vi "_Update Start Up Turbo.vi"(4 "error in (no error)":errorcluster) -> (0 "error Out":errorcluster, 2 "Next InstrState":T1, 3 "Cancel":bool)   [LabVIEW 2018]
uses:
  Type/_RT Instrument State.ctl
  Type/_Pump Parameter.ctl
  Type/_LCD Line1 Msg.ctl
  Type/_LCD Line2 Msg.ctl
  Type/_RW Status.ctl
  Type/_LED States.ctl
  _RT Global.vi
  <vilib>/Utility/error.llb/Error Cluster From Error Code.vi
  <vilib>/rvi/errors/niLvFpgaAdjustHostInterfaceError.vi
  <vilib>/rvi/interface/nirviReadWriteControl/nirviReadWriteControl.xnode
  Type/FPGA Typedef.ctl
  FPGA Bitfiles/FPGA9607.lvbitx
  NiFpgaLv.dll
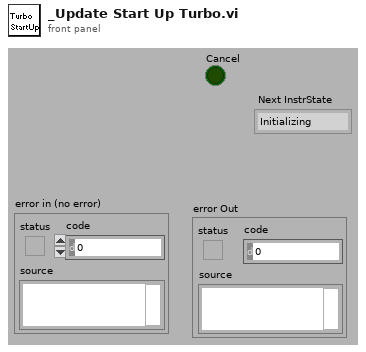
[diagram p1: front panel]
types:
  T1 = typedef "_RT Instrument State.ctl" = enum16{"Initializing", "Mass Spectrometer is Off", "Starting Up", "Turning Power Off", "Going to Standby", "Roughing Pump Ready", "Turning Turbo Off", "Turbo Startup", "Turbopump Ready", "Checking Vacuum", "Going to Ready", "Ready", "Running", "Source Standby", "Lost Communication", "Shutting Down", "Fault", "24V Standby", "Go to 24V Standby", "Turbopump Ready-Waiting"}
  T2 = typedef "_Pump Parameter.ctl" = enum16{"Turn Pump Motor On", "Turn Pump Motor Off", "Read Pump Oil Deficiency", "Read Rotation Switch Point Attained", "Read Ele. Drive Over Temperature", "Read Pump Over Temperature", "Read Set Rotation Speed Attained", "Read Turbopump Accelerates", "Read Actual Rotation Speed in Hz", "Read Motor Current in A", "Read Operating Hours in h", "Read Motor Voltage in V", "Read Motor Power in W", "Set Rotation Speed Switchpoint in %", "Clear Error", "Read Error Code", "Read Bearing Temperature", "Read Hardware Version", "Read Firmware Version", "Read Operating Hours (Drive)", "Read Rotational Speed (rpm)", "Read Power Stage Temperature", "Read Electronics Temperature", "Read Upper Pump Temperature", "Read Motor Temperature", "Read Error Code History, 1", "Read Error Code History, 2", "Read Error Code History, 3", "Read Error Code History, 4", "Read Error Code History, 5", "Read Error Code History, 6", "Read Error Code History, 7", "Read Error Code History, 8", "Read Error Code History, 9", "Read Error Code History, 10"}
  T3 = typedef "_RW Status.ctl" = enum8{"Done", "Do Read", "Do Write", "Set Latch1", "Set Latch2", "Set Latch3", "Set Latch4", "RP ON", "EL ON", "Serial Send", "Set LC Out", "Get LC In", "Read VAC", "Table Test", "Get Interlock", "Do Read2", "Do Write2"}
  T4 = typedef "_LED States.ctl" = enum8{"Idle", "Solid B", "Solid R", "Solid P", "Off B", "Off R", "Off P", "Off BRP", "Off RP", "Flash R&P", "Flash P"}
  T5 = typedef "_LCD Line2 Msg.ctl" = u16
  T6 = typedef "_LCD Line1 Msg.ctl" = u16
  T7 = typedef "_RT Startup Options.ctl" = cluster{"Door":bool, "Curtain":bool, "Pressure":bool, "Turbo":bool, "SysPoll":bool, "GasFlag":bool, "SourceExhaust":bool}
  T8 = typedef "FPGA Typedef.ctl" = refnum<k20>
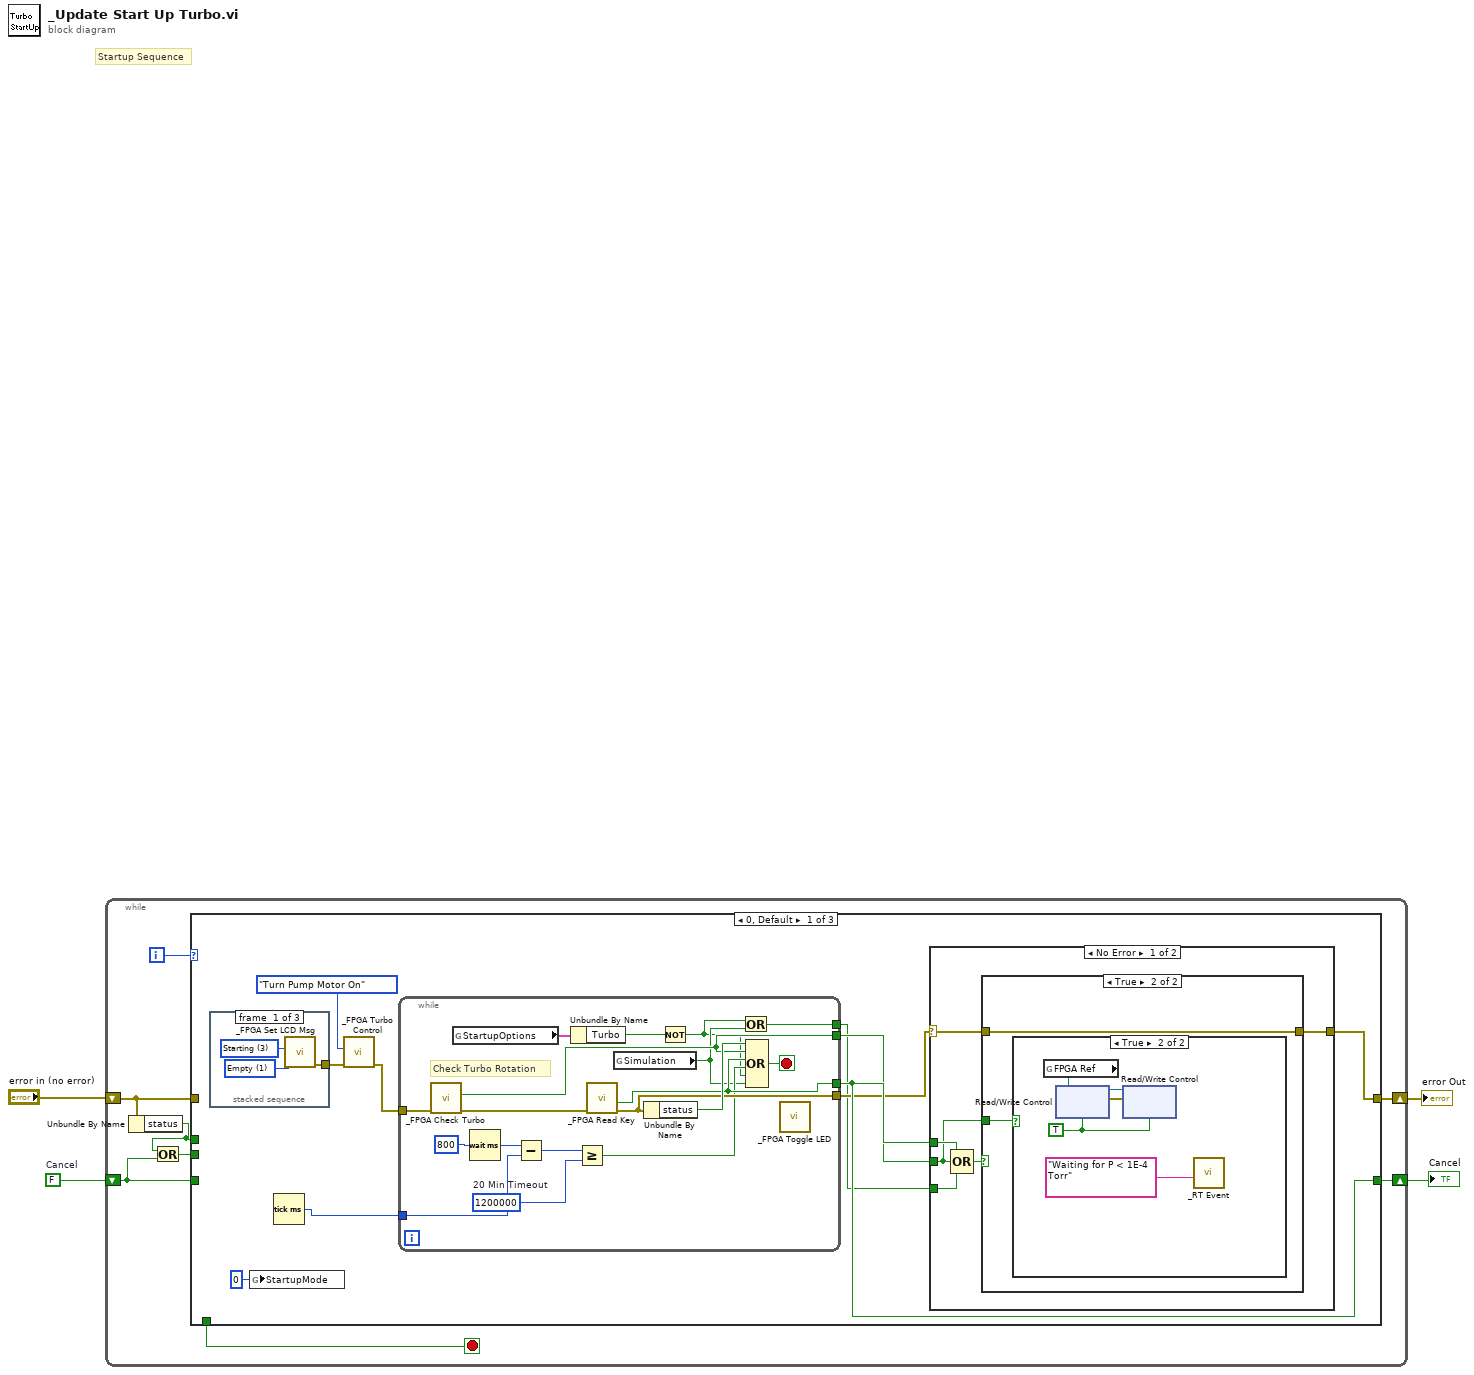
[diagram p0: block diagram]
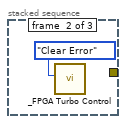
[diagram p2: hidden frame]
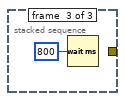
[diagram p3: hidden frame]
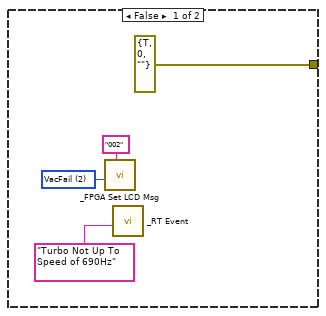
[diagram p4: hidden frame]
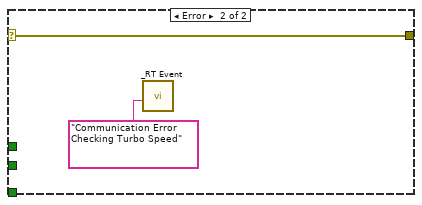
[diagram p6: hidden frame]
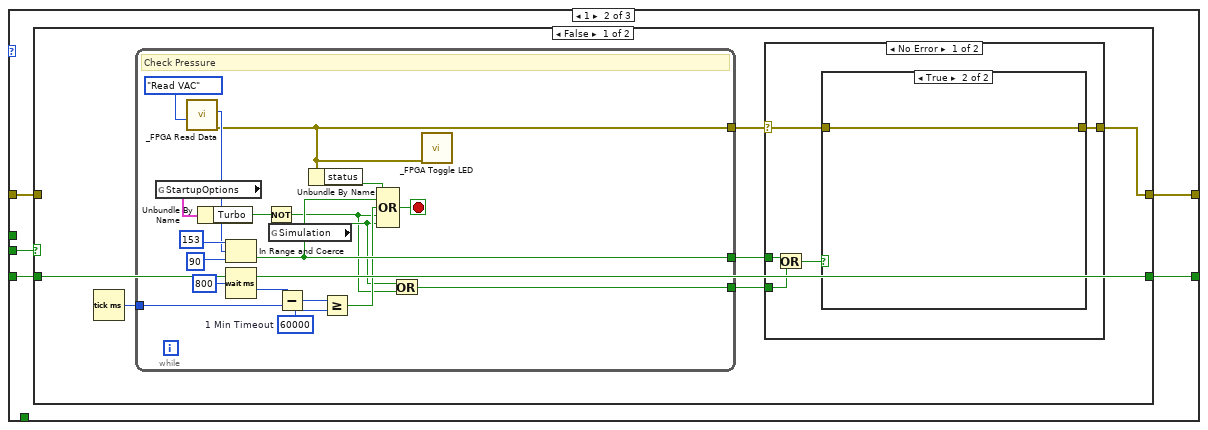
[diagram p7: hidden frame]
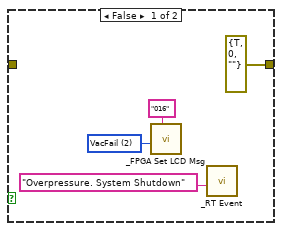
[diagram p8: hidden frame]
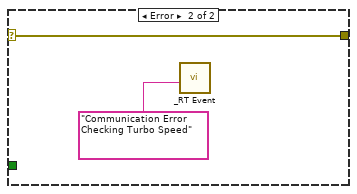
[diagram p9: hidden frame]
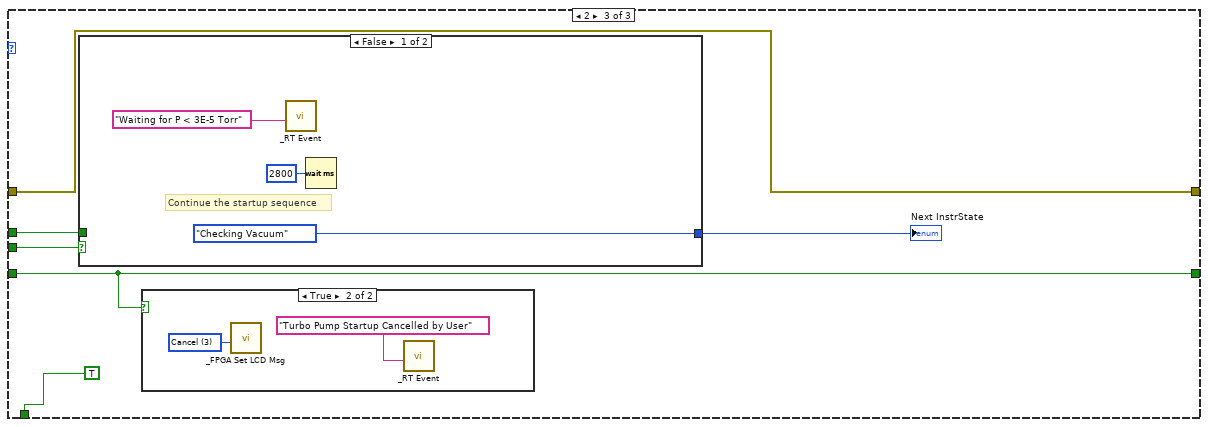
[diagram p11: hidden frame]
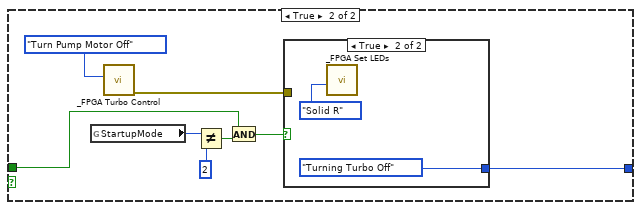
[diagram p12: hidden frame]
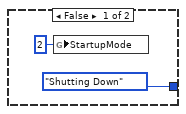
[diagram p13: hidden frame]
diagram:
  w3 = FALSE  # Cancel
  # "Startup Sequence"
  n1 = while {
    shift-right: [w8] -> w2
    shift-left: "error in (no error)" -> [w10]
    shift-right: [w7] -> w1
    shift-left: w3 -> [w9]
    i -> [w12]
    stop <- w6 stop-if-true
    n2 = Unbundle By Name(w10) -> ("status"=w5:bool)
    n3 = Or(x=w5, y=w9) -> (x .or. y?=w11:bool)
    n4 = case shown="0, Default" w12 {
      tunnel: w11 -> [_ w67 w111]
      tunnel: w10 -> [_ w66 w113]
      tunnel: w9 -> [_ w65 w112]
      tunnel: [w22 w69 w113] -> w8
      tunnel: [w21 w68 w112] -> w7
      tunnel: [_ _ TRUE] -> w6
      tunnel: w5 -> [_ _ w109]
      frame 0, Default {
        n5 = stacked-sequence {
          tunnel: [w41 _ _] -> w15
          frame #0 {
            w42 = T5 1 items=["Same", "Empty", "VacFail", "Cancel", "CheckGas", "EleFail", "Probe1Fail", "Probe2Fail", "HeaterFail", "DoorOpen", "CheckComm", "PressStart", "StartRP"] ("Line2Msg (same)")
            w43 = T6 3 items=["Same", "Empty", "Connected", "Starting", "Stopping", "Action", "On", "Service", "Call", "Acquiring", "Source"] ("Line1Msg (same)")
            n6 = call "_FPGA Set LCD Msg.vi"("Line2Msg (same)"=w42, "Line1Msg (same)"=w43) -> ("error out"=w41:errorcluster)  [unwired: 5 in, 2 out]
          }
          frame #1 {
            n7 = call "_FPGA Turbo Control.vi"("Command"=_Pump_Parameter."Clear Error") -> ()  [unwired: 3 in, 6 out]
          }
          frame #2 {
            n8 = Wait (ms)(milliseconds to wait=u32 800) -> ()  [unwired: 1 out]
          }
        }
        n9 = global write "_RT Global.vi" "StartupMode"(u8 0 ("StartupMode")) -> ()
        n10 = Tick Count (ms)() -> (millisecond timer value=w13:u32)
        n11 = call "_FPGA Turbo Control.vi"("error in (no error)"=w15, "Command"=_Pump_Parameter."Turn Pump Motor On") -> ("error out"=w14:errorcluster)  [unwired: 2 in, 5 out]
        n12 = while {
          tunnel: w14 -> [w31]
          tunnel: [w37] -> w20
          tunnel: [w36] -> w21
          tunnel: w13 -> [w32]
          tunnel: [w29] -> w19
          tunnel: [w26] -> w17
          stop <- w40 stop-if-true
          w35 = u32 1200000  # 20 Min Timeout
          # "Check Turbo Rotation"
          n13 = call "_FPGA Check Turbo.vi"("error in"=w31) -> ("error out"=w30:errorcluster, "SpeedOK"=w29:bool)  [unwired: 1 in, 4 out]
          n14 = global read "_RT Global.vi" "StartupOptions"() -> (w25:T7)
          n15 = Wait (ms)(milliseconds to wait=u32 800) -> (millisecond timer value=w33:u32)
          n16 = Subtract(x=w33, y=w32) -> (x-y=w34:u32)
          n17 = Unbundle By Name(w25) -> ("Turbo"=w24:bool)
          n18 = Greater Or Equal?(x=w34, y=w35) -> (x >= y?=w28:bool)
          n19 = call "_FPGA Read Key.vi"("error in (no error)"=w30) -> ("error out"=w37:errorcluster, "Key Pressed"=w36:bool)  [unwired: 3 in, 3 out]
          n20 = global read "_RT Global.vi" "Simulation"() -> (w27:bool)
          n21 = Unbundle By Name(w37) -> ("status"=w39:bool)
          n22 = Not(x=w24) -> (.not. x?=w23:bool)
          n23 = Or(x=w23, y=w27) -> (x .or. y?=w26:bool)
          n24 = Compound Arithmetic op=OR(w39, w29, w36, w28, w23, w27) -> (w40:bool)
          n25 = call "_FPGA Toggle LED.vi"() -> ()  [unwired: 5 in, 4 out]
        }
        n26 = case shown="No Error" w20 {
          selector: w20 -> [w51 w64]
          tunnel: w19 -> [w47 _]
          tunnel: [w50 w64] -> w22
          tunnel: w21 -> [w48 _]
          tunnel: w17 -> [w46 _]
          frame No Error {
            n27 = Compound Arithmetic op=OR(w48, w47, w46) -> (w49:bool)
            n28 = case shown="True" w49 {
              tunnel: [errorcluster {"status"=TRUE, "code"=0, "source"=""} ("error IO") w57] -> w50
              tunnel: w51 -> [_ w57]
              tunnel: w47 -> [_ w56]
              frame False {
                w53 = T5 2 items=["Same", "Empty", "VacFail", "Cancel", "CheckGas", "EleFail", "Probe1Fail", "Probe2Fail", "HeaterFail", "DoorOpen", "CheckComm", "PressStart", "StartRP"] ("Line2Msg (same)")
                n29 = call "_FPGA Set LCD Msg.vi"("ErrNum"="002", "Line2Msg (same)"=w53) -> ()  [unwired: 4 in, 4 out]
                n30 = call "_RT Event.vi"("Event"="Turbo Not Up To      Speed of 690Hz" ("Command")) -> ()  [unwired: 2 in, 5 out]
              }
              frame True {
                n31 = case shown="True" w56 {
                  frame False {
                  }
                  frame True {
                    w62 = TRUE
                    n32 = global read "_RT Global.vi" "FPGA Ref"() -> (w58:T8)
                    n33 = xnode "Read/Write Control"("FPGA VI Reference In"=w58, "FilaB"=w62) -> ("FPGA VI Reference Out"=w60:T8, "error out"=w61:errorcluster)  [unwired: 1 in]
                    n34 = xnode "Read/Write Control"("FPGA VI Reference In"=w60, "error in"=w61, "FilaC"=w62) -> ()  [unwired: 2 out]
                    n35 = call "_RT Event.vi"("Event"="Waiting for P < 1E-4 Torr" ("Command")) -> ()  [unwired: 2 in, 5 out]
                  }
                }
              }
            }
          }
          frame Error {
            n36 = call "_RT Event.vi"("Event"="Communication Error Checking Turbo Speed") -> ()  [unwired: 2 in, 5 out]
          }
        }
      }
      frame 1 {
        n37 = case shown="False" w67 {
          tunnel: [w71 w107] -> w68
          tunnel: [w73 w108] -> w69
          tunnel: w66 -> [_ w108]
          tunnel: w65 -> [w71 w107]
          frame False {
            n38 = Tick Count (ms)() -> (millisecond timer value=w72:u32)
            n39 = while {
              tunnel: [w76] -> w75
              tunnel: w72 -> [w90]
              tunnel: [w88] -> w74
              tunnel: [w80] -> w70
              stop <- w94 stop-if-true
              w84 = u32 60000  # 1 Min Timeout
              # "Check Pressure"
              n40 = global read "_RT Global.vi" "StartupOptions"() -> (w79:T7)
              n41 = call "_FPGA Read Data.vi"("Read Mode (Do Read)"=_RW_Status."Read VAC" ("R/W Status")) -> ("error out"=w76:errorcluster, "Data"=w85:u32)  [unwired: 4 in, 1 out]
              n42 = Unbundle By Name(w79) -> ("Turbo"=w78:bool)
              n43 = In Range and Coerce(upper limit=u32 153, x=w85, lower limit=u32 90 ("y")) -> (In Range?=w88:bool)  [unwired: 1 out]
              n44 = Wait (ms)(milliseconds to wait=u32 800) -> (millisecond timer value=w91:u32)
              n45 = Not(x=w78) -> (.not. x?=w77:bool)
              n46 = global read "_RT Global.vi" "Simulation"() -> (w81:bool)
              n47 = Subtract(x=w91, y=w90) -> (x-y=w83:u32)
              n48 = Unbundle By Name(w76) -> ("status"=w93:bool)
              n49 = Greater Or Equal?(x=w83, y=w84) -> (x >= y?=w82:bool)
              n50 = Compound Arithmetic op=OR(w93, w88, w82, w77, w81) -> (w94:bool)
              n51 = Or(x=w81, y=w77) -> (x .or. y?=w80:bool)
              n52 = call "_FPGA Toggle LED.vi"("error in (no error)"=w76) -> ()  [unwired: 4 in, 4 out]
            }
            n53 = case shown="No Error" w75 {
              selector: w75 -> [w99 w106]
              tunnel: w74 -> [w95 _]
              tunnel: [w98 w106] -> w73
              tunnel: w70 -> [w96 _]
              frame No Error {
                n54 = Or(x=w95, y=w96) -> (x .or. y?=w97:bool)
                n55 = case shown="True" w97 {
                  tunnel: [errorcluster {"status"=TRUE, "code"=0, "source"=""} ("error IO") w104] -> w98
                  tunnel: w99 -> [_ w104]
                  frame False {
                    w101 = T5 2 items=["Same", "Empty", "VacFail", "Cancel", "CheckGas", "EleFail", "Probe1Fail", "Probe2Fail", "HeaterFail", "DoorOpen", "CheckComm", "PressStart", "StartRP"] ("Line2Msg (same)")
                    n56 = call "_FPGA Set LCD Msg.vi"("ErrNum"="016", "Line2Msg (same)"=w101) -> ()  [unwired: 4 in, 4 out]
                    n57 = call "_RT Event.vi"("Event"="Overpressure. System Shutdown" ("Command")) -> ()  [unwired: 2 in, 5 out]
                  }
                  frame True {
                  }
                }
              }
              frame Error {
                n58 = call "_RT Event.vi"("Event"="Communication Error Checking Turbo Speed") -> ()  [unwired: 2 in, 5 out]
              }
            }
          }
          frame True {
          }
        }
      }
      frame 2 {
        n59 = case shown="False" w111 {
          tunnel: [_RT_Instrument_State."Checking Vacuum" ("Next InstrState") w124] -> w110
          tunnel: w109 -> [_ w120]
          frame False {
            # "Continue the startup sequence"
            n60 = call "_RT Event.vi"("Event"="Waiting for P < 3E-5 Torr" ("Command")) -> ()  [unwired: 2 in, 5 out]
            n61 = Wait (ms)(milliseconds to wait=u32 2800) -> ()  [unwired: 1 out]
          }
          frame True {
            n62 = global read "_RT Global.vi" "StartupMode"() -> (w123:u8)
            n63 = call "_FPGA Turbo Control.vi"("Command"=_Pump_Parameter."Turn Pump Motor Off") -> ("error out"=w118:errorcluster)  [unwired: 3 in, 5 out]
            n64 = Not Equal?(x=w123, y=u8 2) -> (x != y?=w121:bool)
            n65 = And(x=w120, y=w121) -> (x .and. y?=w119:bool)
            n66 = case shown="True" w119 {
              tunnel: [_RT_Instrument_State."Shutting Down" ("Next InstrState") _RT_Instrument_State."Turning Turbo Off" ("Next InstrState")] -> w124
              tunnel: w118 -> [_ _]
              frame False {
                n67 = global write "_RT Global.vi" "StartupMode"(u8 2 ("StartupMode")) -> ()
              }
              frame True {
                n68 = call "_FPGA Set LEDs.vi"("LED Command"=_LED_States."Solid R") -> ()  [unwired: 3 in, 4 out]
              }
            }
          }
        }
        "Next InstrState" <- w110
        n69 = case shown="True" w112 {
          frame False {
          }
          frame True {
            w131 = T5 3 items=["Same", "Empty", "VacFail", "Cancel", "CheckGas", "EleFail", "Probe1Fail", "Probe2Fail", "HeaterFail", "DoorOpen", "CheckComm", "PressStart", "StartRP"] ("Line2Msg (same)")
            n70 = call "_FPGA Set LCD Msg.vi"("Line2Msg (same)"=w131) -> ()  [unwired: 6 in, 3 out]
            n71 = call "_RT Event.vi"("Event"="Turbo Pump Startup Cancelled by User" ("Command")) -> ()  [unwired: 2 in, 5 out]
          }
        }
      }
    }
  }
  "error Out" <- w2
  "Cancel" <- w1
